vi "Dryer Read.vi"(0 "Com Chan":u8, 7 "Dryer Status Serial Data In":T1, 11 "error in (no error)":errorcluster) -> (4 "Dryer Status Serial Data":T1, 6 "Read Buffer":string, 8 "Log String":string, 15 "error out":errorcluster)   [LabVIEW 2012]
uses:
  Dryer Com Port Info.ctl
  Dryer Status Ctrl.ctl
  GEA2 Driver/GEA2 Dryer Interface Ctrl.ctl
  Globals Wilt.vi
panel:
  out "x-y 3":u32
  out "x-y 2":u32
  out "x-y":u32
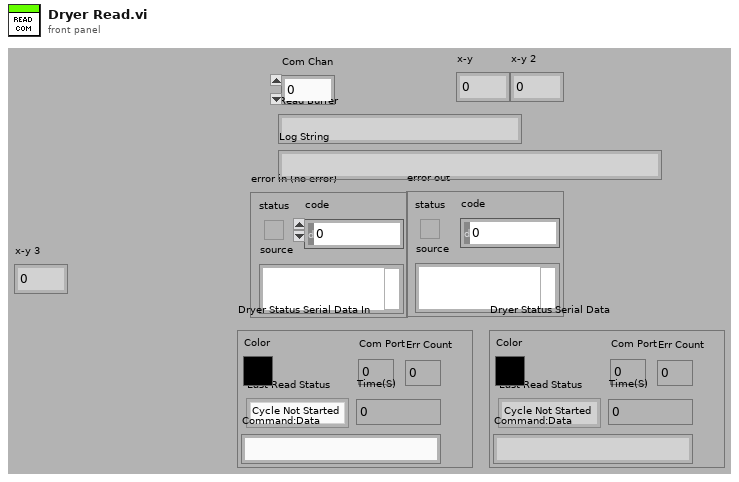
[diagram p1: front panel]
types:
  T1 = typedef "Dryer Com Port Info.ctl" = cluster{"Color":u32, "Last Read Status":T2, "Command:Data":string, "Com Port":u8, "Time(S)":dbl, "Err Count":u32}
  T2 = typedef "Dryer Status Ctrl.ctl" = enum16{"Cycle Not Started", "Cycle Running", "Paused", "Cycle Completed", "Eval Mode Entered", "Err"}
  T3 = typedef "GEA2 Dryer Interface Ctrl.ctl" = enum16{"Init Com Port", "SendCMD", "ReadPort", "Close Port", "Simulate Diag Data", "Simulate Dryer", "Send WILT Startup CMDs", "Send Continue CMD", "Read Continuous"}
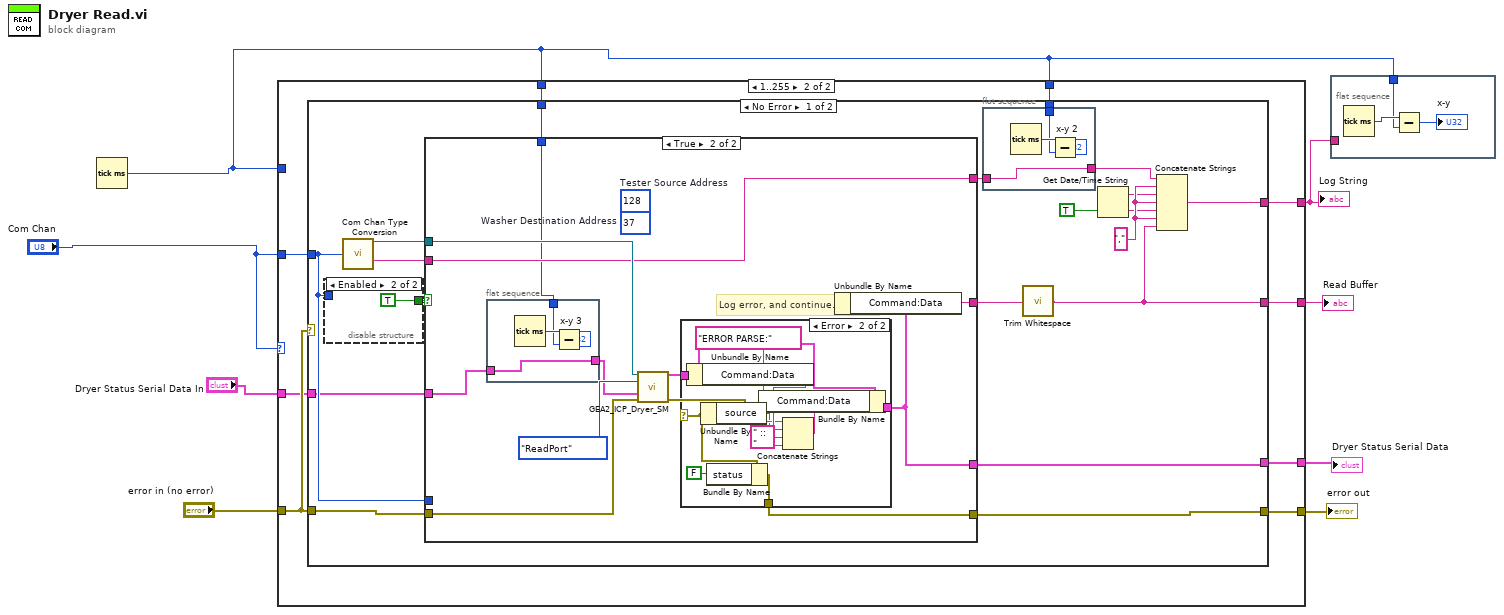
[diagram p0: block diagram]
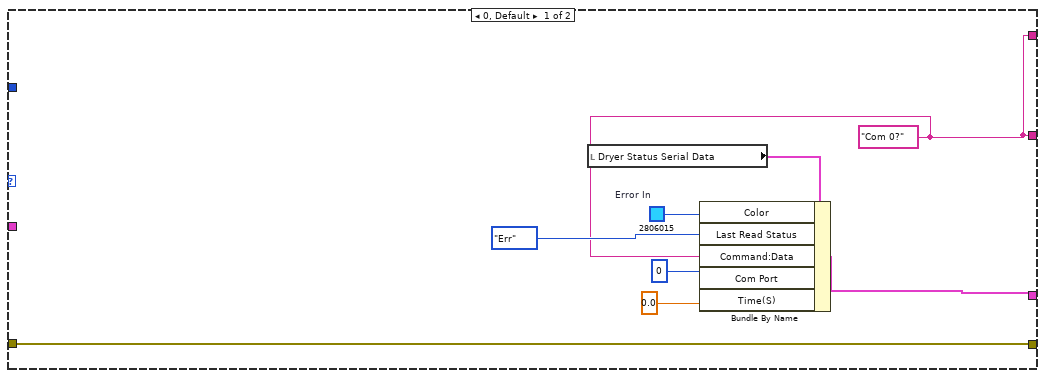
[diagram p2: hidden frame]
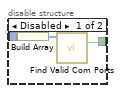
[diagram p3: hidden frame]
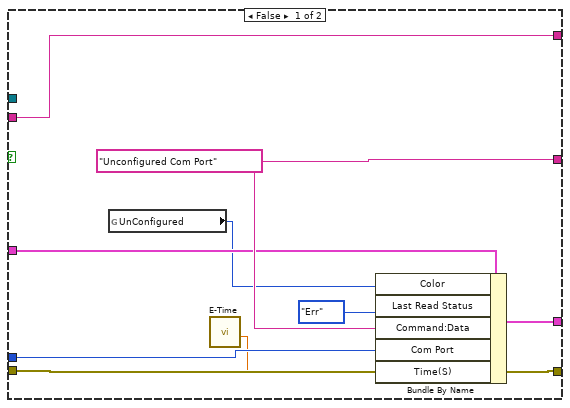
[diagram p4: hidden frame]
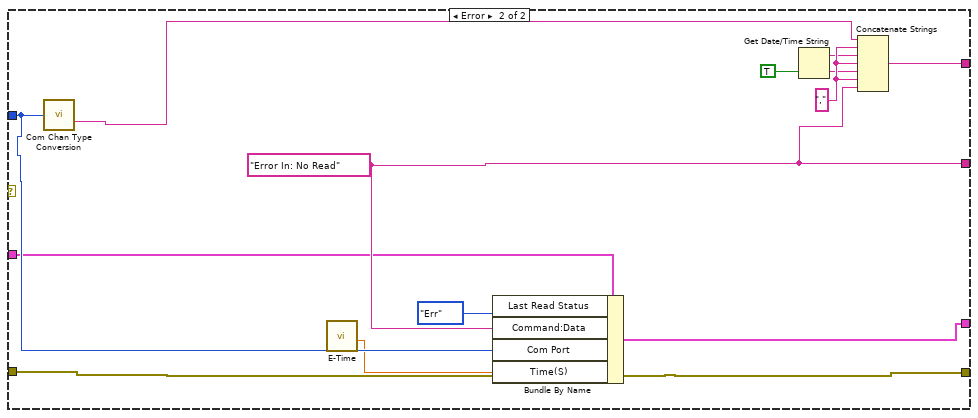
[diagram p6: hidden frame]
diagram:
  n1 = Tick Count (ms)() -> (millisecond timer value=w1:u32)
  n2 = case shown="1..255" "Com Chan" {
    tunnel: "Com Chan" -> [_ w25]
    tunnel: [w16 w24] -> w8
    tunnel: "error in (no error)" -> [w16 w23]
    tunnel: [w12 w22] -> w2
    tunnel: [w12 w21] -> w5
    tunnel: [w9 w20] -> w4
    tunnel: "Dryer Status Serial Data In" -> [_ w19]
    tunnel: w1 -> [_ _]
    tunnel: w1 -> [_ w18]
    tunnel: w1 -> [_ w17]
    frame 0, Default {
      w13 = u32 2806015  # Error In
      w12 = "Com 0?" ("ASCII Data")
      n3 = local read "Dryer Status Serial Data"() -> (w15:T1)
      n4 = Bundle By Name(cluster=w15, "Color"=w13, "Last Read Status"=Dryer_Status_Ctrl."Err" ("Status"), "Command:Data"=w12, "Com Port"=u8 0, "Time(S)"=0.0) -> (w9:T1)
    }
    frame 1..255 {
      n5 = case shown="No Error" w23 {
        tunnel: w25 -> [w35 w96]
        tunnel: [w44 w102] -> w24
        tunnel: w23 -> [w43 w102]
        tunnel: [w34 w93] -> w22
        tunnel: [w26 w92] -> w21
        tunnel: [w33 w91] -> w20
        tunnel: w19 -> [w32 w90]
        tunnel: w18 -> [w29 _]
        tunnel: w17 -> [w28 _]
        frame No Error {
          w39 = "," ("string")
          n6 = disable-structure shown="Enabled" {
            disable-tunnel: [w46 TRUE ("Found?")] -> w40
            disable-tunnel: w35 -> [w45 _]
            frame Disabled {
              n7 = Build Array(w45) -> (w47:u8[])
              n8 = call "Find Valid Com Ports.vi"("Valid Com Port List(100,2:56)"=w47) -> ("Found?"=w46:bool)  [unwired: 13 in, 1 out]
            }
            frame Enabled {
            }
          }
          n9 = call "Com Chan Type Conversion.vi"("Com Chan"=w35) -> ("VISA resource name"=w42:refnum<visa-resource-name>, "Com Text"=w41:string)  [unwired: 11 in, 2 out]
          n10 = case shown="True" w40 {
            tunnel: [w56 w62] -> w44
            tunnel: w43 -> [w56 w73]
            tunnel: w42 -> [_ w72]
            tunnel: w41 -> [w61 w69]
            tunnel: [w60 w64] -> w33
            tunnel: [w58 w70] -> w27
            tunnel: [w61 w69] -> w30
            tunnel: w35 -> [w59 _]
            tunnel: w32 -> [w54 w68]
            tunnel: w28 -> [_ w66]
            frame False {
              w58 = "Unconfigured Com Port" ("ASCII Data")
              n11 = global read "Globals Wilt.vi" "UnConfigured"() -> (w53:u32)
              n12 = call "E-Time.vi"() -> ("Elapsed Time (sec)"=w55:dbl)  [unwired: 9 in, 2 out]
              n13 = Bundle By Name(cluster=w54, "Color"=w53, "Last Read Status"=Dryer_Status_Ctrl."Err" ("Status"), "Command:Data"=w58, "Com Port"=w59, "Time(S)"=w55) -> (w60:T1)
            }
            frame True {
              (unwired) u8 128  # Tester Source Address
              (unwired) u8 37  # Washer Destination Address
              # "Log error, and continue."
              n14 = flat-sequence {
                tunnel: [w89] -> w67
                tunnel: w68 -> [w89]
                tunnel: w66 -> [w87]
                frame #0 {
                  n15 = Tick Count (ms)() -> (millisecond timer value=w88:u32)
                  n16 = Subtract(x=w88, y=w87) -> (x-y=→"x-y 3":u32)
                }
              }
              n17 = call "GEA2_ICP_Dryer_SM.vi"("ComPort"=w72, "Mode"=GEA2_Dryer_Interface_Ctrl."ReadPort", "Dryer Status Serial Data In"=w67, "Error In"=w73) -> ("Dryer Status Serial Data Out"=w63:T1, "Error Out"=w65:errorcluster)  [unwired: 6 in, 4 out]
              n18 = case shown="Error" w65 {
                selector: w65 -> [w74 w77]
                tunnel: [w75 w84] -> w64
                tunnel: w63 -> [w75 w85]
                tunnel: [w74 w78] -> w62
                frame No Error {
                }
                frame Error {
                  n19 = Unbundle By Name(w85) -> ("Command:Data"=w82:string)
                  n20 = Unbundle By Name(w77) -> ("source"=w80:string)
                  n21 = Bundle By Name(cluster=w77, "status"=FALSE) -> (w78:errorcluster)
                  n22 = Concatenate Strings("ERROR PARSE:" ("string"), w80, " :: " ("string"), w82) -> (w83:string)
                  n23 = Bundle By Name(cluster=w85, "Command:Data"=w83) -> (w84:T1)
                }
              }
              n24 = Unbundle By Name(w64) -> ("Command:Data"=w70:string)
            }
          }
          n25 = flat-sequence {
            tunnel: [w52] -> w31
            tunnel: w30 -> [w52]
            tunnel: w29 -> [w50]
            frame #0 {
              n26 = Tick Count (ms)() -> (millisecond timer value=w51:u32)
              n27 = Subtract(x=w51, y=w50) -> (x-y=→"x-y 2":u32)
            }
          }
          n28 = call <vilib>:"Trim Whitespace.vi"("string"=w27) -> ("trimmed string"=w26:string)  [unwired: 1 in]
          n29 = Get Date/Time String(want seconds? (F)=TRUE) -> (date string=w37:string, time string=w38:string)  [unwired: 2 in]
          n30 = Concatenate Strings(w31, w39, w37, w39, w38, w39, w26) -> (w34:string)
        }
        frame Error {
          w92 = "Error In: No Read" ("ASCII Data")
          w101 = "," ("string")
          n31 = call "Com Chan Type Conversion.vi"("Com Chan"=w96) -> ("Com Text"=w97:string)  [unwired: 11 in, 3 out]
          n32 = call "E-Time.vi"() -> ("Elapsed Time (sec)"=w94:dbl)  [unwired: 9 in, 2 out]
          n33 = Bundle By Name(cluster=w90, "Last Read Status"=Dryer_Status_Ctrl."Err" ("Status"), "Command:Data"=w92, "Com Port"=w96, "Time(S)"=w94) -> (w91:T1)
          n34 = Get Date/Time String(want seconds? (F)=TRUE) -> (date string=w99:string, time string=w100:string)  [unwired: 2 in]
          n35 = Concatenate Strings(w97, w101, w99, w101, w100, w101, w92) -> (w93:string)
        }
      }
    }
  }
  "error out" <- w8
  "Log String" <- w2
  "Read Buffer" <- w5
  "Dryer Status Serial Data" <- w4
  n36 = flat-sequence {
    tunnel: w2 -> [_]
    tunnel: w1 -> [w104]
    frame #0 {
      n37 = Tick Count (ms)() -> (millisecond timer value=w105:u32)
      n38 = Subtract(x=w105, y=w104) -> (x-y=→"x-y":u32)
    }
  }
